vi "Hash File with SHA-256.vi"(6 "Blocksize (1Mb)":u32=1048576 min=64 step=64, 8 "error In":errorcluster, 11 "Path to Hash":path) -> (0 "error Out":errorcluster, 3 "Hash String":string)   [LabVIEW 2018, in "SHA256.lvlib"]
doc: "Calculates the SHA-256 hash for a file on dosc."
uses:
  SHA256.lvlib
  chi.vi
  Sigma1.vi
  ma.vi
  Sigma0.vi
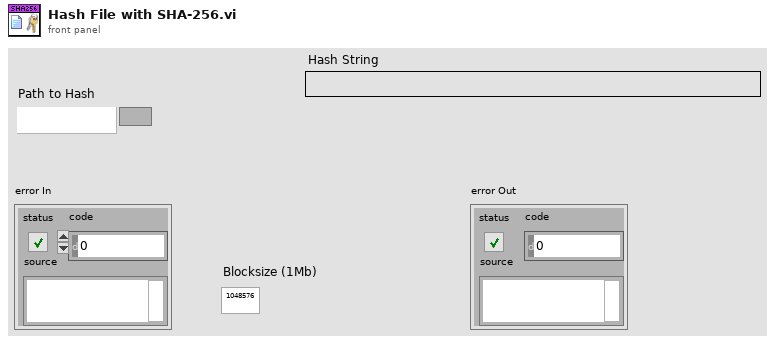
[diagram p1: front panel]
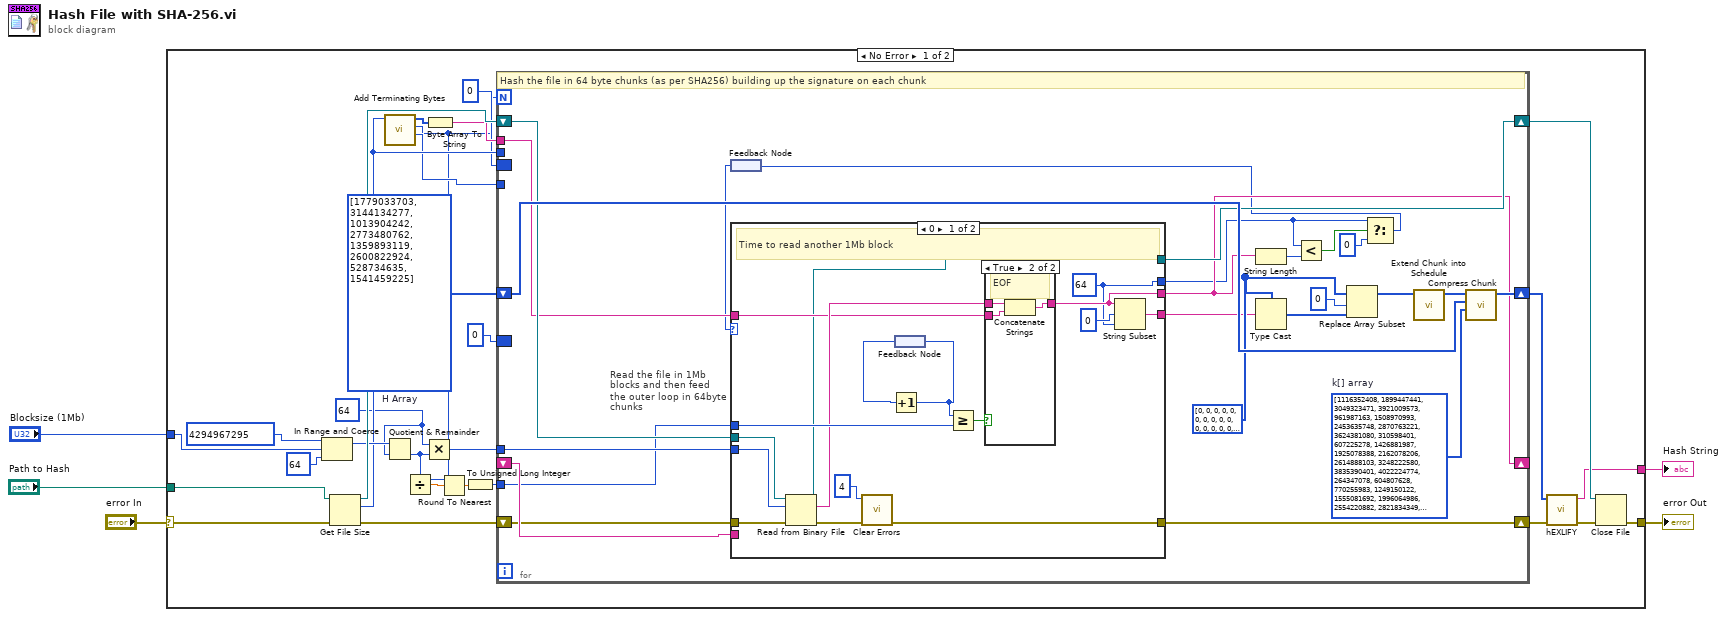
[diagram p0: block diagram]
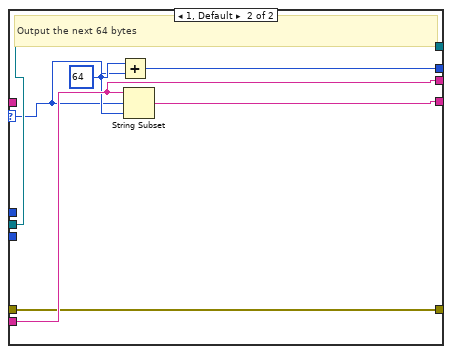
[diagram p3: hidden frame]
diagram:
  n1 = case shown="No Error" "error In" {
    selector: "error In" -> [w33 w86]
    tunnel: [w23 w86] -> w5
    tunnel: [w22 _] -> w4
    tunnel: "Blocksize (1Mb)" -> [w20 _]
    tunnel: "Path to Hash" -> [w17 _]
    frame No Error {
      w12 = u32 64 ("y")
      w29 = u32[] [1779033703, 3144134277, 1013904242, 2773480762, 1359893119, 2600822924, 528734635, 1541459225]  # H Array
      n2 = In Range and Coerce(upper limit=u32 4294967295, x=w20, lower limit=u32 64) -> (coerced(x)=w21:u32)  [unwired: 1 out]
      n3 = Get File Size(file=w17, error in=w33) -> (refnum out=w32:refnum<file>, size (in bytes)=w15:i64, 0:w27:errorcluster)
      n4 = call "Add Terminating Bytes.vi"("Size of Data"=w15) -> ("Extra bytes"=w13:i32, "Number of Chunks"=w10:i32, "Array"=w31:u8[])  [unwired: 8 in]
      n5 = Quotient & Remainder(x=w21, y=w12) -> (floor(x/y)=w9:u32)  [unwired: 1 out]
      n6 = Divide(x=w10, y=w9) -> (x/y=w8:dbl)
      n7 = Multiply(x=w12, y=w9) -> (x*y=w19:u32)
      n8 = Byte Array To String(unsigned byte array=w31) -> (string=w30:string)
      n9 = Round To Nearest(number=w8) -> (nearest integer value=w7:dbl)
      n10 = To Unsigned Long Integer(number=w7) -> (unsigned 32bit integer=w6:u32)
      n11 = for {
        N: w10 -> [_]
        shift-right: [w47] -> w25
        shift-left: w32 -> [w46]
        shift-right: [w41] -> _
        shift-left: _ -> [w57]
        tunnel: w30 -> [w43]
        shift-right: [w51] -> w28
        shift-left: w29 -> [w50]
        shift-right: [w48] -> w26
        shift-left: w27 -> [w49]
        tunnel: w19 -> [w44]
        tunnel: w15 -> [_]
        border: 0 ("f") -> [_]
        tunnel: w13 -> [_]
        border: u32 0 -> [_]
        tunnel: w6 -> [w34]
        w45 = u32[] [0, 0, 0, 0, 0, 0, 0, 0, 0, 0, 0, 0, 0, 0, 0, 0, 0, 0, 0, 0, 0, 0, 0, 0, 0, 0, 0, 0, 0, 0, 0, 0, 0, 0, 0, 0, 0, 0, 0, 0, 0, 0, 0, 0, 0, 0, 0, 0, 0, 0, 0, 0, 0, 0, 0, 0, 0, 0, 0, 0, 0, 0, 0, 0]
        w56 = u32[] [1116352408, 1899447441, 3049323471, 3921009573, 961987163, 1508970993, 2453635748, 2870763221, 3624381080, 310598401, 607225278, 1426881987, 1925078388, 2162078206, 2614888103, 3248222580, 3835390401, 4022224774, 264347078, 604807628, 770255983, 1249150122, 1555081692, 1996064986, 2554220882, 2821834349, 2952996808, 3210313671, 3336571891, 3584528711, 113926993, 338241895, 666307205, 773529912, 1294757372, 1396182291, 1695183700, 1986661051, 2177026350, 2456956037, 2730485921, 2820302411, 3259730800, 3345764771, 3516065817, 3600352804, 4094571909, 275423344, 430227734, 506948616, 659060556, 883997877, 958139571, 1322822218, 1537002063, 1747873779, 1955562222, 2024104815, 2227730452, 2361852424, 2428436474, 2756734187, 3204031479, 3329325298]  # k[] array
        # "Hash the file in 64 byte chunks (as per SHA256) building up the signature on each chunk"
        n12 = feedback #1() -> (w35:i32)
        n13 = case "Read the file in 1Mb blocks and then feed\nthe outer loop in 64byte chunks" shown="0" w35 {
          selector: w35 -> [_ w79]
          tunnel: [w63 w85] -> w41
          tunnel: w57 -> [_ w85]
          tunnel: [w71 w84] -> w42
          tunnel: w49 -> [w70 w83]
          tunnel: [w61 w83] -> w48
          tunnel: [w58 w82] -> w47
          tunnel: w46 -> [w69 w82]
          tunnel: w44 -> [w68 _]
          tunnel: w34 -> [w67 _]
          tunnel: w43 -> [w64 _]
          tunnel: [w62 w80] -> w38
          frame 0 {
            w62 = 64 ("length (rest)")
            # "Time to read another 1Mb block"
            n14 = Read from Binary File(8:w70, 10:w68, 11:w69) -> (0:w74:errorcluster, 2:w65:string, 3:w58:refnum<file>)  [unwired: 3 in, 1 out]
            n15 = call <vilib>:"Clear Errors.vi"("error in (no error)"=w74, "specific error code to clear (0: all)"=4) -> ("error out"=w61:errorcluster)  [unwired: 4 in, 1 out]
            n16 = feedback #2() -> (w60:u32)
            n17 = Increment(x=w60) -> (x+1=w59:u32)
            n18 = feedback-in #2(w59) -> ()
            n19 = Greater Or Equal?(x=w59, y=w67) -> (x >= y?=w66:bool)
            n20 = case shown="True" w66 {
              tunnel: w65 -> [w75 w78]
              tunnel: w64 -> [_ w77]
              tunnel: [w75 w76] -> w63
              frame False {
              }
              frame True {
                # "EOF"
                n21 = Concatenate Strings(w78, w77) -> (w76:string)
              }
            }
            n22 = String Subset(string=w63, offset (0)=0, length (rest)=w62) -> (substring=w71:string)
          }
          frame 1, Default {
            w81 = 64
            # "Output the next 64 bytes"
            n23 = Add(x=w81, y=w79) -> (x+y=w80:i32)
            n24 = String Subset(string=w85, offset (0)=w79, length (rest)=w81) -> (substring=w84:string)
          }
        }
        n25 = String Length(string=w41) -> (length=w40:i32)
        n26 = Type Cast(type=w45, x=w42) -> (*(type *) &x=w52:u32[])
        n27 = Less?(x=w38, y=w40) -> (x < y?=w39:bool)
        n28 = Replace Array Subset(array=w45, new element=w52, index=0) -> (w54:u32[])
        n29 = Select(t=w38, s=w39, f=0) -> (s? t:f=w36:i32)
        n30 = feedback-in #1(w36) -> ()
        n31 = call "Extend Chunk into Schedule.vi"("Array in"=w54) -> ("Array out"=w55:u32[])  [unwired: 10 in]
        n32 = call "Compress Chunk.vi"("Key Array"=w56, "Hash In"=w50, "Data Array In"=w55) -> ("Hash Out"=w51:u32[])  [unwired: 8 in]
      }
      n33 = call "hEXLIFY.vi"("error in (no error)"=w26, "H Array"=w28) -> ("error out"=w24:errorcluster, "String"=w22:string)  [unwired: 8 in]
      n34 = Close File(refnum=w25, error in=w24) -> (error out=w23:errorcluster)  [unwired: 1 out]
    }
    frame Error {
    }
  }
  "Hash String" <- w4
  "error Out" <- w5
